vi "Time Message Events.vi"(8 "error in (no error)":errorcluster, 10 "Debug Mode":bool, 11 "Message in":T1={"Command"="", "Data"=variant(string ""), "ID"=""}) -> (0 "error out":errorcluster, 2 "time (ms)":u32, 3 "Message out":T1={"Command"="", "Data"=variant(string ""), "ID"=""})   [LabVIEW 2019, in "RemoteControl.lvclass"]
uses:
  RemoteControl.lvclass
  Typedefs/Message--Cluster.ctl
  <vilib>/Utility/Data Type/Type Definitions/Data Type.ctl
  <vilib>/Utility/Data Type/NI_Data Type.lvlib
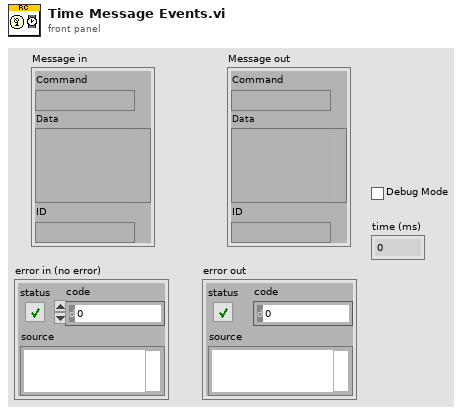
[diagram p1: front panel]
types:
  T1 = typedef "RemoteControl.lvclass/Message--Cluster.ctl" = cluster{"Command":string, "Data":variant, "ID":string}
  T2 = typedef "NI_Data Type.lvlib/Data Type.ctl" = enum8{"Invalid Type", "Void", "I8", "I16", "I32", "I64", "U8", "U16", "U32", "U64", "Single Float", "Double Float", "Extended Float", "Single Complex", "Double Complex", "Extended Complex", "Enum U8", "Enum U16", "Enum U32", "Enum U64", "Single Float With Unit", "Double Float With Unit", "Extended Float With Unit", "Single Complex with Unit", "Double Complex with Unit", "Extended Complex with Unit", "Boolean", "String", "Path", "Picture", "Tag", "Array", "Cluster", "Variant", "LV Variant", "Waveform", "Timestamp", "Digital Waveform", "Digital Data", "ExpressData", "Refnum", "External Data", "VI", "Poly VI", "LabVIEW Class Instance", "Fixed Point", "Set Collection", "Map Collection"}
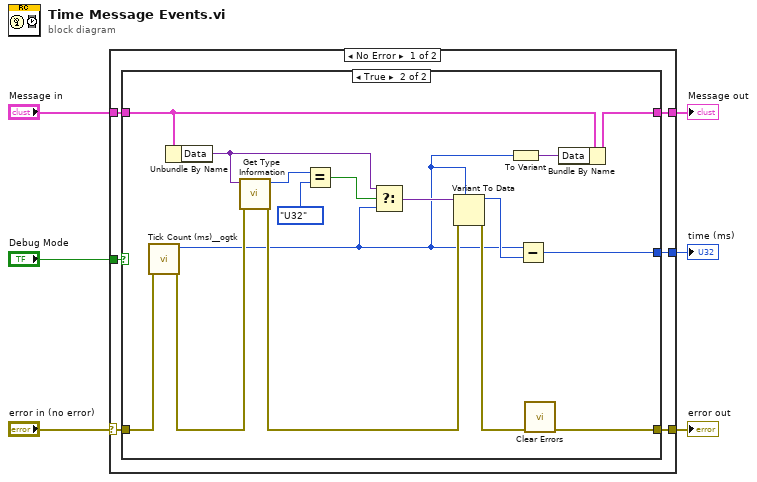
[diagram p0: block diagram]
diagram:
  n1 = case shown="No Error" "error in (no error)" {
    selector: "error in (no error)" -> [w7 w32]
    tunnel: [w12 w32] -> w6
    tunnel: [w11 _] -> w5
    tunnel: [w10 w31] -> w4
    tunnel: "Message in" -> [w9 w31]
    tunnel: "Debug Mode" -> [w8 _]
    frame No Error {
      n2 = case shown="True" w8 {
        tunnel: [w13 w23] -> w12
        tunnel: w7 -> [w13 w28]
        tunnel: [_ w27] -> w11
        tunnel: [w14 w26] -> w10
        tunnel: w9 -> [w14 w25]
        frame False {
        }
        frame True {
          n3 = call <userlib>:"Tick Count (ms)__ogtk.vi"("error in (no error)"=w28) -> ("error out"=w22:errorcluster, "millisecond timer value"=w15:u32)  [unwired: 9 in]
          n4 = Unbundle By Name(w25) -> ("Data"=w18:variant)
          n5 = call <vilib>:"Get Type Information.vi"("error in (no error)"=w22, "variant"=w18) -> ("error out"=w21:errorcluster, "type"=w19:T2)  [unwired: 5 in, 3 out]
          n6 = Equal?(x=w19, y=Data_Type."U32" ("Type")) -> (x = y?=w17:bool)
          n7 = Select(t=w18, s=w17, f=w15) -> (s? t:f=w16:variant)
          n8 = Variant To Data(error in=w21, type=w15, Variant=w16) -> (data=w30:u32, error out=w29:errorcluster)
          n9 = To Variant(anything=w15) -> (Variant=w24:variant)
          n10 = Subtract(x=w15, y=w30) -> (x-y=w27:u32)
          n11 = call <vilib>:"Clear Errors.vi"("error in (no error)"=w29) -> ("error out"=w23:errorcluster)  [unwired: 5 in, 1 out]
          n12 = Bundle By Name(cluster=w25, "Data"=w24) -> (w26:T1)
        }
      }
    }
    frame Error {
    }
  }
  "error out" <- w6
  "Message out" <- w4
  "time (ms)" <- w5
